vi "Read.vi"(6 "Append Index":i32, 8 "error in (no error)":errorcluster, 11 "Data.TDMS":refnum<class "Data.TDMS.lvclass">) -> (0 "error out":errorcluster, 1 "Notes":string, 2 "Data (Dictionary)":T1[](array[typedef]), 3 "Data.TDMS out":refnum<class "Data.TDMS.lvclass">, 5 "Path out":path)   [LabVIEW 2019, in "Data.TDMS.lvclass"]
uses:
  Data.TDMS.lvclass
  Data/Data.lvclass
  Data/Typedefs/Dictionary--cluster.ctl
  Data/Typedefs/Operation--enum.ctl
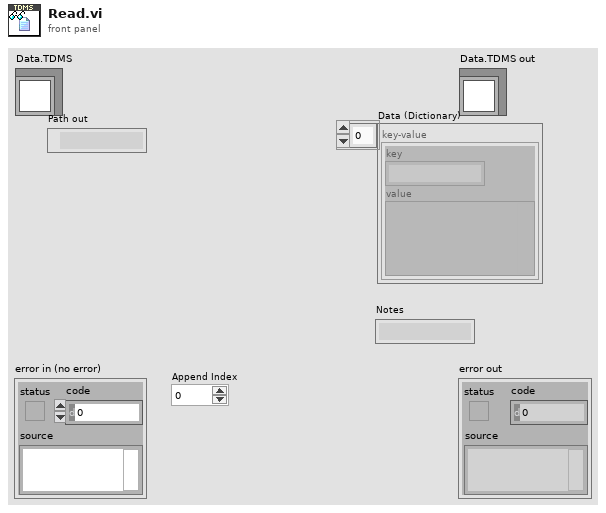
[diagram p1: front panel]
types:
  T1 = typedef "Data.lvclass/Dictionary--cluster.ctl" = cluster{"key":string, "value":variant}
  T2 = typedef "Data.lvclass/Operation--enum.ctl" = enum16{"Read", "Write", "Write + Append"}
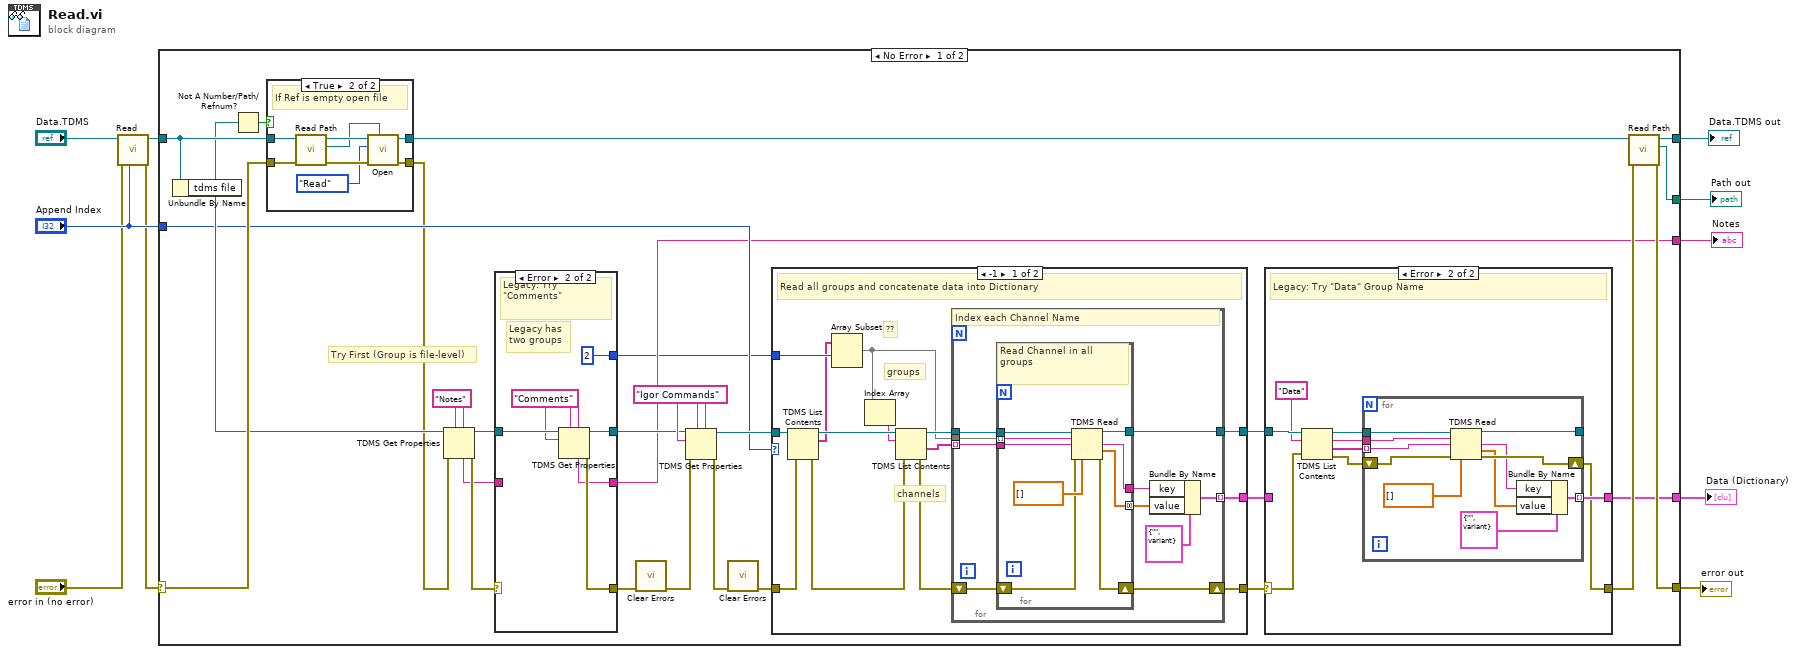
[diagram p0: block diagram]
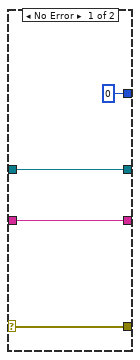
[diagram p3: hidden frame]
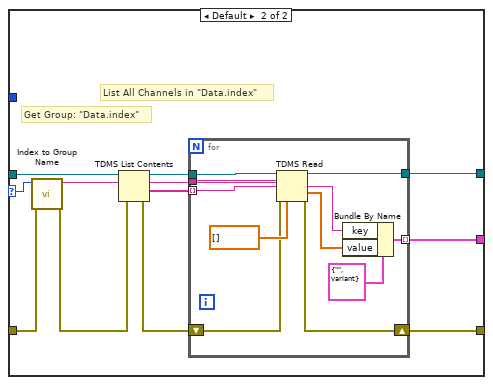
[diagram p4: hidden frame]
diagram:
  n1 = call-parent "Read.vi"("Append Index"="Append Index", "error in (no error)"="error in (no error)", "Data Save in"="Data.TDMS") -> ("error out"=w1:errorcluster, "Data Save out"=w4:refnum<class "Data.TDMS.lvclass">)  [unwired: 4 in, 3 out]
  n2 = case shown="No Error" w1 {
    selector: w1 -> [w31 w136]
    tunnel: w4 -> [w33 w135]
    tunnel: [w36 w135] -> w10
    tunnel: [w35 w136] -> w9
    tunnel: [w37 _] -> w8
    tunnel: "Append Index" -> [w23 _]
    tunnel: [w12 _] -> w7
    tunnel: [w19 _] -> w6
    frame No Error {
      w27 = "Notes" ("group name")
      w30 = "Igor Commands" ("attrib name")
      # "Try First (Group is file-level)"
      n3 = Unbundle By Name(w33) -> ("tdms file"=w25:refnum<k34>)
      n4 = Not A Number/Path/Refnum?(number/path/refnum=w25) -> (NaN/Path/Refnum?=w34:bool)
      n5 = case shown="True" w34 {
        tunnel: w33 -> [w39 w47]
        tunnel: [w39 w48] -> w32
        tunnel: [w40 w44] -> w17
        tunnel: w31 -> [w40 w43]
        frame False {
        }
        frame True {
          # "If Ref is empty open file"
          n6 = call "Read Path.vi"("error in (no error)"=w43, "Data Save"=w47) -> ("error out"=w46:errorcluster, "Path"=w41:path, "Data Save out"=w45:refnum<class "Data.TDMS.lvclass">)  [unwired: 7 in]
          n7 = call-dynamic "Open.vi"("Path"=w41, "error in (no error)"=w46, "Operation"=Operation--enum."Read", "Data.TDMS in"=w45) -> ("error out"=w44:errorcluster, "Data.TDMS out"=w48:refnum<class "Data.TDMS.lvclass">)  [unwired: 6 in]
        }
      }
      n8 = TDMS Get Properties(5:w27, 7:w27, 8:w17, 11:w25) -> (0:w29:errorcluster, 3:w26:refnum<k34>, 4:w28:string)  [unwired: 2 in, 3 out]
      n9 = case shown="Error" w29 {
        selector: w29 -> [w52 _]
        tunnel: [w52 w58] -> w16
        tunnel: w28 -> [w51 _]
        tunnel: [w51 w57] -> w12
        tunnel: w26 -> [w50 w56]
        tunnel: [w50 w55] -> w24
        tunnel: [0 ("index") 2 ("index")] -> w11
        frame No Error {
        }
        frame Error {
          w54 = "Comments" ("group name")
          # "Legacy has\ntwo groups"
          # "Legacy: Try \"Comments\""
          n10 = TDMS Get Properties(5:w54, 7:w54, 10:w54, 11:w56) -> (0:w58:errorcluster, 3:w55:refnum<k34>, 4:w57:string)  [unwired: 2 in, 3 out]
        }
      }
      n11 = call <vilib>:"Clear Errors.vi"("error in (no error)"=w16) -> ("error out"=w15:errorcluster)  [unwired: 5 in, 1 out]
      n12 = TDMS Get Properties(5:w30, 7:w30, 8:w15, 10:w30, 11:w24) -> (0:w14:errorcluster, 3:w38:refnum<k34>)  [unwired: 1 in, 4 out]
      n13 = call <vilib>:"Clear Errors.vi"("error in (no error)"=w14) -> ("error out"=w13:errorcluster)  [unwired: 5 in, 1 out]
      n14 = case shown="-1" w23 {
        selector: w23 -> [_ w97]
        tunnel: w38 -> [w71 w103]
        tunnel: w13 -> [w62 w96]
        tunnel: [w65 w99] -> w20
        tunnel: [w72 w98] -> w22
        tunnel: [w61 w94] -> w18
        tunnel: w11 -> [w60 _]
        frame -1 {
          # "??"
          # "groups"
          # "channels"
          # "Read all groups and concatenate data into Dictionary"
          n15 = TDMS List Contents(4:w62, 7:w71) -> (0:w67:errorcluster, 2:w59:string[], 3:w70:refnum<k34>)  [unwired: 1 in, 1 out]
          n16 = Array Subset(array=w59, index=w60) -> (w63:string[])  [unwired: 1 in]
          n17 = Index Array(array=w63) -> (element=w64:string)  [unwired: 1 in]
          n18 = TDMS List Contents(4:w67, 6:w64, 7:w70) -> (0:w66:errorcluster, 1:w69:string[], 3:w68:refnum<k34>)  [unwired: 1 out]
          n19 = for {
            tunnel: [w75] -> w65 mode=indexing
            tunnel: w68 -> [w81]
            shift-right: [w82] -> w72
            shift-left: w66 -> [w74]
            tunnel: w63 -> [w80]
            tunnel: w69 -> [w79] mode=indexing
            tunnel: [w73] -> w61
            # "Index each Channel Name"
            n20 = for {
              shift-right: [w83] -> w82
              shift-left: w74 -> [w84]
              tunnel: w79 -> [w89]
              tunnel: w80 -> [w90] mode=indexing
              tunnel: w81 -> [w91]
              tunnel: [w87] -> w78 mode=concatenating
              tunnel: [w86] -> w77
              tunnel: [w85] -> w73
              # "Read Channel in all groups"
              n21 = TDMS Read(0:w91, 5:w90, 7:w89, 11:w84, 12:dbl[] [] ("array type (2D Dbl)")) -> (4:w85:refnum<k34>, 8:w86:string, 10:w87:dbl[], 15:w83:errorcluster)  [unwired: 3 in, 2 out]
            }
            n22 = Bundle By Name(cluster=T1 {"key"="", "value"=variant} ("key-value"), "key"=w77, "value"=w78) -> (w75:T1)
          }
        }
        frame Default {
          # "List All Channels in \"Data.index\""
          # "Get Group: \"Data.index\""
          n23 = call "Index to Group Name.vi"("error in (no error)"=w96, "Append Index"=w97) -> ("error out"=w92:errorcluster, "group name in (Untitled)"=w95:string)  [unwired: 8 in]
          n24 = TDMS List Contents(4:w92, 6:w95, 7:w103) -> (0:w93:errorcluster, 1:w100:string[], 2:w101:string, 3:w102:refnum<k34>)
          n25 = for {
            shift-right: [w104] -> w98
            shift-left: w93 -> [w105]
            tunnel: w100 -> [w106] mode=indexing
            tunnel: w101 -> [w112]
            tunnel: [w111] -> w99 mode=indexing
            tunnel: w102 -> [w113]
            tunnel: [w107] -> w94
            n26 = TDMS Read(0:w113, 5:w112, 7:w106, 11:w105, 12:dbl[] [] ("array type (2D Dbl)")) -> (4:w107:refnum<k34>, 10:w108:dbl[], 15:w104:errorcluster)  [unwired: 3 in, 3 out]
            n27 = Bundle By Name(cluster=T1 {"key"="", "value"=variant} ("key-value"), "key"=w106, "value"=w108) -> (w111:T1)
          }
        }
      }
      n28 = case shown="Error" w22 {
        selector: w22 -> [w115 w119]
        tunnel: [w115 w116] -> w21
        tunnel: w20 -> [w114 _]
        tunnel: [w114 w117] -> w19
        tunnel: w18 -> [_ w120]
        frame No Error {
        }
        frame Error {
          # "Legacy: Try \"Data\" Group Name"
          n29 = TDMS List Contents(4:w119, 6:"Data" ("group name"), 7:w120) -> (0:w122:errorcluster, 1:w124:string[], 2:w123:string, 3:w121:refnum<k34>)
          n30 = for {
            shift-right: [w132] -> w116
            shift-left: w122 -> [w134]
            tunnel: w124 -> [w125] mode=indexing
            tunnel: w123 -> [w131]
            tunnel: [w130] -> w117 mode=indexing
            tunnel: w121 -> [w133]
            tunnel: [w126] -> _
            n31 = TDMS Read(0:w133, 5:w131, 7:w125, 11:w134, 12:dbl[] [] ("array type (2D Dbl)")) -> (4:w126:refnum<k34>, 10:w127:dbl[], 15:w132:errorcluster)  [unwired: 3 in, 3 out]
            n32 = Bundle By Name(cluster=T1 {"key"="", "value"=variant} ("key-value"), "key"=w125, "value"=w127) -> (w130:T1)
          }
        }
      }
      n33 = call "Read Path.vi"("error in (no error)"=w21, "Data Save"=w32) -> ("error out"=w35:errorcluster, "Path"=w37:path, "Data Save out"=w36:refnum<class "Data.TDMS.lvclass">)  [unwired: 7 in]
    }
    frame Error {
    }
  }
  "error out" <- w9
  "Data.TDMS out" <- w10
  "Path out" <- w8
  "Data (Dictionary)" <- w6
  "Notes" <- w7
